vi "comparison_square_root.vi"() -> ()   [LabVIEW 2019]
panel:
  in  "karekok sayısı":dbl
  out "sqrt(x)":dbl
  out "Numeric":i32
  in  "stop":bool
  out "c":dbl
  in  "b":dbl
  in  "a":dbl
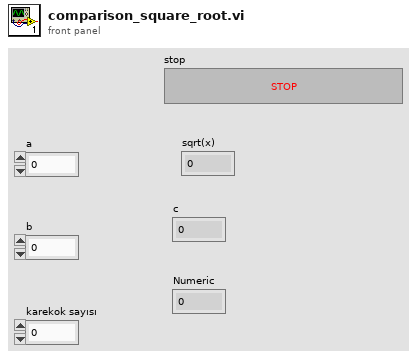
[diagram p1: front panel]
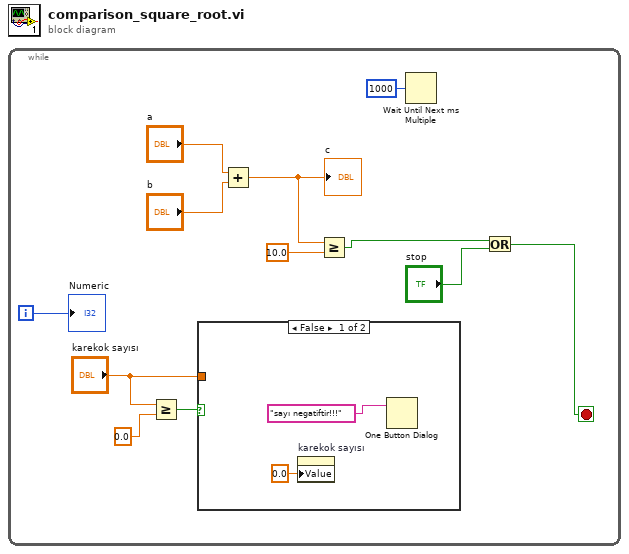
[diagram p0: block diagram]
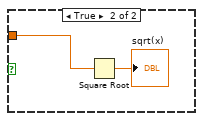
[diagram p2: hidden frame]
diagram:
  n1 = while {
    i -> [w10]
    stop <- w1 stop-if-true
    n2 = Greater Or Equal?(x="karekok sayısı", y=0.0) -> (x >= y?=w3:bool)
    n3 = case shown="False" w3 {
      tunnel: "karekok sayısı" -> [_ w15]
      frame False {
        n4 = property on="karekok sayısı" class="DigNum (strict)"("Value"=0.0 ("karekok sayısı")) -> ()  [unwired: 2 in, 2 out]
        n5 = One Button Dialog(message="sayı negatiftir!!!") -> ()  [unwired: 1 in, 1 out]
      }
      frame True {
        n6 = Square Root(x=w15) -> (sqrt(x)=→"sqrt(x)":dbl)
      }
    }
    n7 = Add(x="a", y="b") -> (x+y=w7:dbl)
    "c" <- w7
    n8 = Greater Or Equal?(x=w7, y=10.0) -> (x >= y?=w6:bool)
    n9 = Wait Until Next ms Multiple(millisecond multiple=u32 1000) -> ()  [unwired: 1 out]
    n10 = Or(x=w6, y="stop") -> (x .or. y?=w1:bool)
    "Numeric" <- w10
  }
